vi "simple digital from wf params.vi"(1 "waveform params":T1, 2 "number of samples":i32) -> (0 "digital waveform":digitalwaveform(waveform))   [LabVIEW 2015]
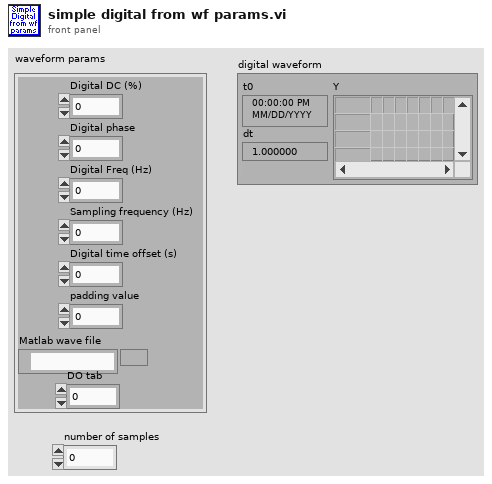
[diagram p1: front panel]
types:
  T1 = cluster{"Digital DC (%)":dbl, "Digital phase":dbl, "Digital Freq (Hz)":dbl, "Sampling frequency (Hz)":dbl, "Digital time offset (s) ":dbl, "padding value":dbl, "Matlab wave file":path, "DO tab":dbl}
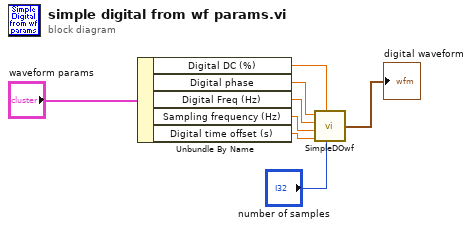
[diagram p0: block diagram]
diagram:
  n1 = Unbundle By Name("waveform params") -> ("Digital DC (%)"=w1:dbl, "Digital phase"=w2:dbl, "Digital Freq (Hz)"=w3:dbl, "Sampling frequency (Hz)"=w4:dbl, "Digital time offset (s)"=w5:dbl)
  n2 = call "SimpleDOwf.vi"("size(s)"="number of samples", "Digital DC (%)"=w1, "Digital time offset"=w5, "Sampling frequency (Hz)"=w4, "Digital Freq (Hz)"=w3, "Digital phase (s)"=w2) -> ("digital waveform"=→"digital waveform":digitalwaveform)
